vi "new itc and dmm file.vi"() -> ()   [LabVIEW 2009]
panel:
  out "Sensor Resistance":dynamicdata(graph)
  out "Sensors Temperature":dynamicdata(graph)
  out "Resistance":dynamicdata(graph)
  out "Temperature":dynamicdata(graph)
  out "Measurement":bool caption="Taken"
  in  "stop":bool
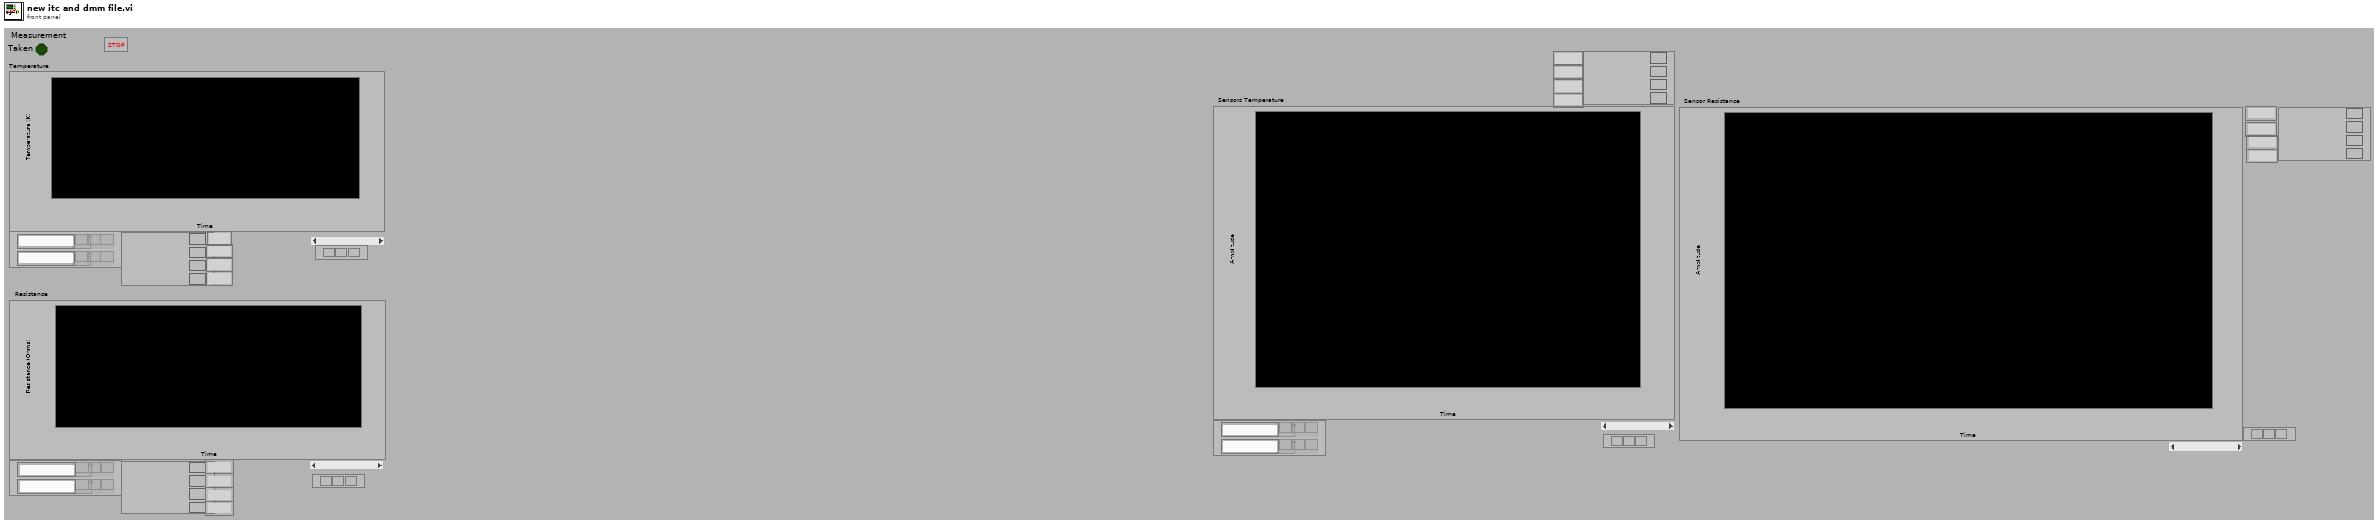
[diagram p1: front panel]
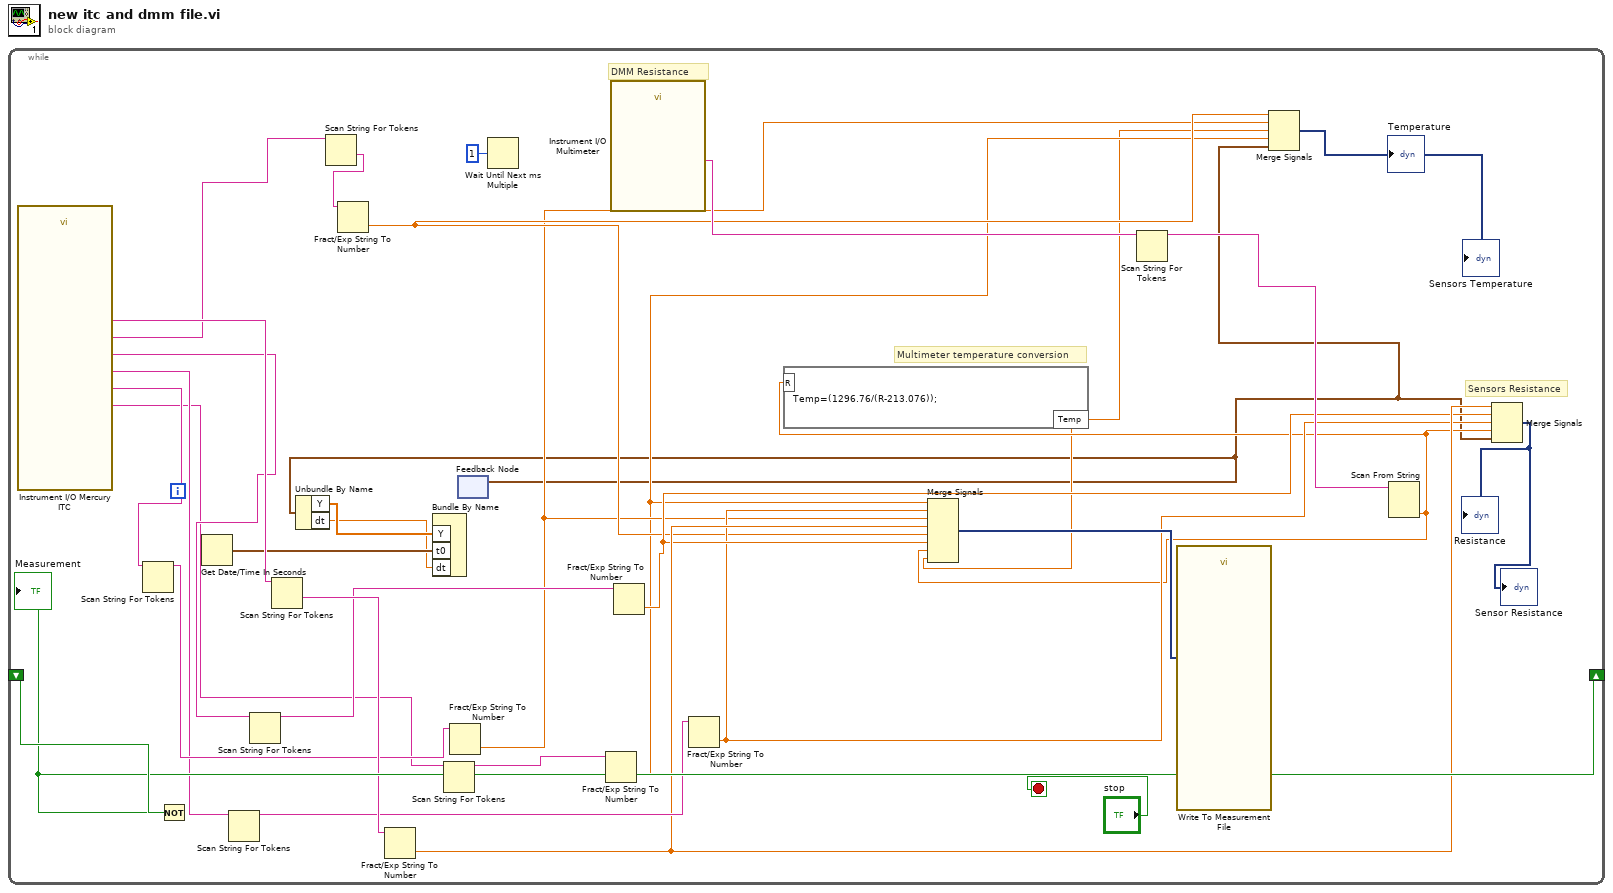
[diagram p0: block diagram]
diagram:
  n1 = while {
    shift-right: [w33] -> _
    shift-left: _ -> [w34]
    stop <- "stop" stop-if-true
    # "DMM Resistance"
    # "Sensors Resistance"
    # "Multimeter temperature conversion"
    n2 = call "Instrument I/O Mercury ITC"() -> ("CCS Resistance"=w22:string, "CCS Temperature"=w20:string, "Allen Bradley Temperature"=w24:string, "Allen Bradley Resistance"=w26:string, "Cernox Temp"=w30:string, "Cernox Resistance"=w32:string)  [unwired: 20 in, 2 out]
    n3 = Scan String For Tokens(9:w24) -> (3:w23:string)  [unwired: 5 in, 3 out]
    n4 = Not(x=w34) -> (.not. x?=w33:bool)
    "Measurement" <- w33
    n5 = Get Date/Time In Seconds() -> (seconds since 1Jan1904=w27:timestamp)
    n6 = Scan String For Tokens(9:w22) -> (3:w21:string)  [unwired: 5 in, 3 out]
    n7 = Scan String For Tokens(9:w26) -> (3:w25:string)  [unwired: 5 in, 3 out]
    n8 = Scan String For Tokens(9:w32) -> (1:w31:string)  [unwired: 5 in, 3 out]
    n9 = Scan String For Tokens(9:w30) -> (1:w28:string)  [unwired: 5 in, 3 out]
    n10 = Fract/Exp String To Number(string=w28) -> (number=w11:dbl)  [unwired: 3 in, 1 out]
    n11 = Fract/Exp String To Number(string=w31) -> (number=w15:dbl)  [unwired: 3 in, 1 out]
    n12 = Scan String For Tokens(9:w20) -> (3:w19:string)  [unwired: 5 in, 3 out]
    n13 = Fract/Exp String To Number(string=w23) -> (number=w10:dbl)  [unwired: 3 in, 1 out]
    n14 = feedback #1() -> (w3:waveform(dbl))  [unwired: 1 in]
    n15 = Unbundle By Name(w3) -> ("Y"=w6:dbl[], "dt"=w5:dbl)
    n16 = Bundle By Name("Y"=w6, "t0"=w27, "dt"=w5) -> (w4:waveform(dbl))  [unwired: 1 in]
    n17 = Wait Until Next ms Multiple(millisecond multiple=u32 1) -> ()  [unwired: 1 out]
    n18 = Fract/Exp String To Number(string=w19) -> (number=w9:dbl)  [unwired: 3 in, 1 out]
    n19 = call "Instrument I/O Multimeter"() -> ("Sample rate"=w16:string)  [unwired: 26 in, 1 out]
    n20 = Fract/Exp String To Number(string=w25) -> (number=w14:dbl)  [unwired: 3 in, 1 out]
    n21 = Fract/Exp String To Number(string=w21) -> (number=w13:dbl)  [unwired: 3 in, 1 out]
    n22 = Scan String For Tokens(9:w16) -> (3:w17:string)  [unwired: 5 in, 3 out]
    n23 = Scan From String(input string=w17) -> (output 1=w12:dbl)  [unwired: 4 in, 3 out]
    n24 = formula code="Temp=(1296.76/(R-213.076));"("R"=w12) -> ("Temp"=w8:dbl)
    n25 = Merge Signals(w9, w13, w10, w15, w11, w14, w12, w8) -> (w29:dynamicdata)
    n26 = call "Write To Measurement File"("Signals"=w29) -> ()  [unwired: 16 in, 3 out]
    n27 = Merge Signals(w11, w10, w8, w9, w3) -> (→"Temperature" →"Sensors Temperature":dynamicdata)
    n28 = Merge Signals(w15, w14, w13, w12, w3) -> (→"Resistance" →"Sensor Resistance":dynamicdata)
  }
